vi "RCServoStart.vi"(0 "Device Info":T2={"Serial Number"=-1, "Channel"=0, "Port"=0}, 1 "Engaged":bool=TRUE, 2 "Target Position":dbl, 5 "RCServo Initialization Data":T1={"Velocity Limit"=60.0, "Acceleration"=90.0, "Min PW"=550.0, "Max PW"=2350.0, "Max Position"=180.0, "Min Position"=0.0, "Speed Ramping State"=TRUE}, 11 "error in (no error)":errorcluster, 12 "Connection":u16(ring) items=["No Preference", "Remote", "Local"], 13 "Timeout (mSec)":i32=5000) -> (4 "Phidget ID":u64, 6 "Serial Number Return":i32, 10 "Attached?":bool, 15 "error out":errorcluster)   [LabVIEW 2020, in "Phidget RC Servo.lvlib"]
doc: "${RCServo:StartHeader}"
uses:
  <instrlib>/Phidgets/Phidget RC Servo/Phidget RC Servo.lvlib
  <instrlib>/Phidgets/Phidget Common/Phidget Common.lvlib
panel:
  # "Enabled\n\nDisabled"
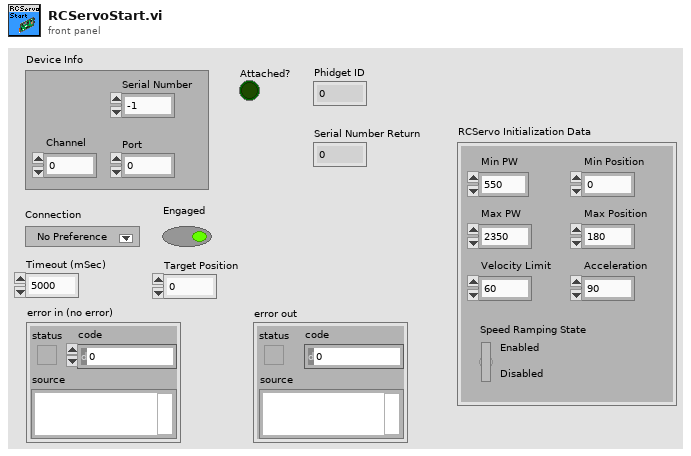
[diagram p1: front panel]
types:
  T1 = cluster{"Velocity Limit":dbl, "Acceleration":dbl, "Min PW":dbl, "Max PW":dbl, "Max Position":dbl, "Min Position":dbl, "Speed Ramping State":bool}
  T2 = cluster{"Serial Number":i32, "Channel":i32, "Port":i32}
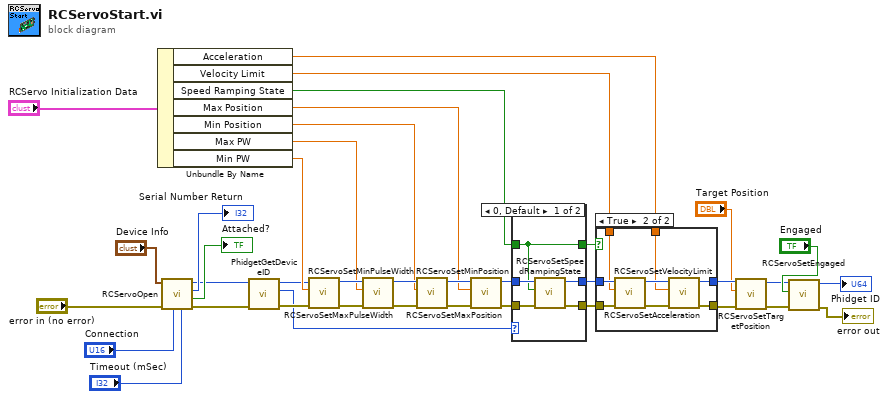
[diagram p0: block diagram]
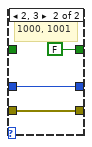
[diagram p2: hidden frame]
diagram:
  n1 = Unbundle By Name("RCServo Initialization Data") -> ("Acceleration"=w19:dbl, "Velocity Limit"=w20:dbl, "Speed Ramping State"=w2:bool, "Max Position"=w24:dbl, "Min Position"=w25:dbl, "Max PW"=w26:dbl, "Min PW"=w27:dbl)
  n2 = call <instrlib>:"RCServoOpen.vi"("Timeout (mSec)"="Timeout (mSec)", "Connection"="Connection", "error in"="error in (no error)", "Device Info"="Device Info") -> ("error out"=w7:errorcluster, "Attached?"=→"Attached?":bool, "Serial Number Return"=→"Serial Number Return":i32, "Phidget ID"=w6:u64)  [unwired: 4 in]
  n3 = call <instrlib>:"PhidgetGetDeviceID.vi"("error in (no error)"=w7, "Device In"=w6) -> ("error out"=w4:errorcluster, "Devie IDs"=w3:u32, "Device Out"=w5:u64)  [unwired: 6 in]
  n4 = call <instrlib>:"RCServoSetMinPulseWidth.vi"("error in (no error)"=w4, "Min Pulse Width"=w27, "Device In"=w5) -> ("error out"=w31:errorcluster, "Device Out"=w34:u64)  [unwired: 6 in]
  n5 = call <instrlib>:"RCServoSetMaxPulseWidth.vi"("error in (no error)"=w31, "Max Pulse Width"=w26, "Device In"=w34) -> ("error out"=w30:errorcluster, "Device Out"=w33:u64)  [unwired: 6 in]
  n6 = call <instrlib>:"RCServoSetMinPosition.vi"("error in (no error)"=w30, "MinPosition"=w25, "Device In"=w33) -> ("error out"=w29:errorcluster, "Device Out"=w32:u64)  [unwired: 6 in]
  n7 = call <instrlib>:"RCServoSetMaxPosition.vi"("error in (no error)"=w29, "Max Position"=w24, "Device In"=w32) -> ("error out"=w21:errorcluster, "Device Out"=w22:u64)  [unwired: 6 in]
  n8 = case shown="0, Default" w3 {
    tunnel: w22 -> [w43 w45]
    tunnel: w21 -> [w42 w44]
    tunnel: [w41 w45] -> w18
    tunnel: [w40 w44] -> w17
    tunnel: w2 -> [w39 _]
    tunnel: [w39 FALSE ("Speed Ramping State")] -> w1
    frame 0, Default {
      n9 = call <instrlib>:"RCServoSetSpeedRampingState.vi"("error in (no error)"=w42, "Speed Ramping State"=w39, "Device In"=w43) -> ("error out"=w40:errorcluster, "Device Out"=w41:u64)  [unwired: 6 in]
    }
    frame 2, 3 {
      # "1000, 1001"
    }
  }
  n10 = case shown="True" w1 {
    tunnel: w20 -> [_ w49]
    tunnel: w19 -> [_ w54]
    tunnel: w18 -> [w48 w53]
    tunnel: w17 -> [w47 w52]
    tunnel: [w48 w51] -> w11
    tunnel: [w47 w50] -> w12
    frame False {
    }
    frame True {
      n11 = call <instrlib>:"RCServoSetVelocityLimit.vi"("error in (no error)"=w52, "Velocity Limit"=w49, "Device In"=w53) -> ("error out"=w55:errorcluster, "Device Out"=w56:u64)  [unwired: 6 in]
      n12 = call <instrlib>:"RCServoSetAcceleration.vi"("error in (no error)"=w55, "Acceleration"=w54, "Device In"=w56) -> ("error out"=w50:errorcluster, "Device Out"=w51:u64)  [unwired: 6 in]
    }
  }
  n13 = call <instrlib>:"RCServoSetTargetPosition.vi"("error in (no error)"=w12, "Target Position"="Target Position", "Device In"=w11) -> ("error out"=w8:errorcluster, "Device Out"=w9:u64)  [unwired: 6 in]
  n14 = call <instrlib>:"RCServoSetEngaged.vi"("error in (no error)"=w8, "Engaged"="Engaged", "Device In"=w9) -> ("error out"=→"error out":errorcluster, "Device Out"=→"Phidget ID":u64)  [unwired: 6 in]
